vi "Clear_Lines.vi"(10 "inputArray":bool[][](array[boolean])) -> (1 "outputArray":bool[][](array[boolean]), 3 "lines":dbl)   [LabVIEW 2015]
panel:
  in  "count":dbl
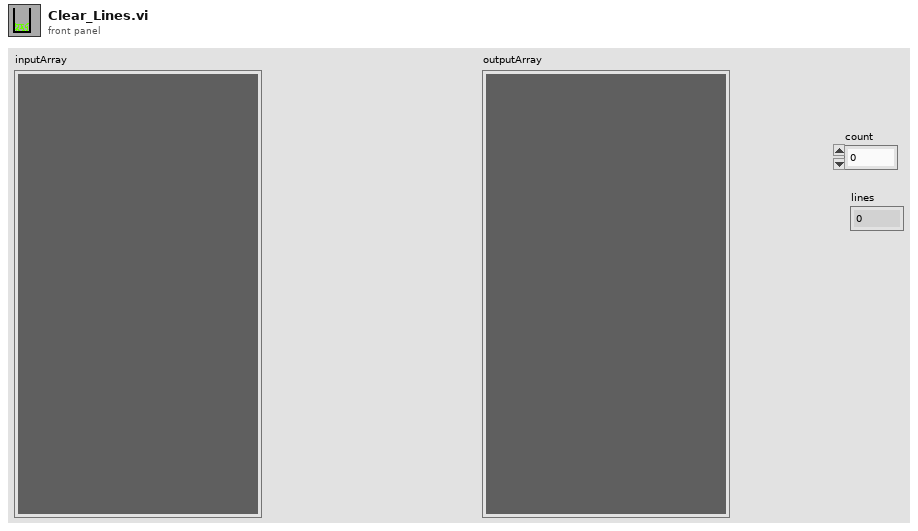
[diagram p1: front panel]
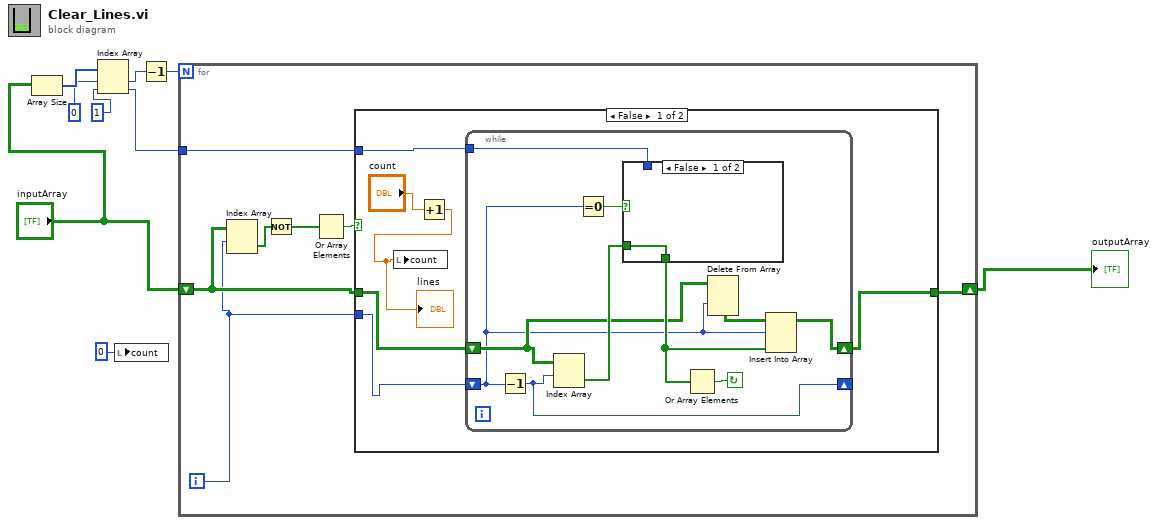
[diagram p0: block diagram]
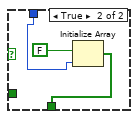
[diagram p2: hidden frame]
diagram:
  n1 = Array Size(array="inputArray") -> (size(s)=w8:i32[])
  n2 = Index Array(array=w8, index #1=0, index #2=1) -> (element #1=w6:i32, element #2=w4:i32)
  n3 = local write "count"(0) -> ()
  n4 = Decrement(x=w6) -> (x-1=w2:i32)
  n5 = for {
    N: w2 -> [_]
    shift-right: [w10] -> w3
    shift-left: "inputArray" -> [w13]
    tunnel: w4 -> [w14]
    i -> [w12]
    n6 = Index Array(array=w13, index (row)=w12) -> (element=w11:bool[])  [unwired: 1 in]
    n7 = Not(x=w11) -> (.not. x?=w16:bool[])
    n8 = Or Array Elements(Boolean array=w16) -> (logical OR=w15:bool)
    n9 = case shown="False" w15 {
      tunnel: w12 -> [w21 _]
      tunnel: w13 -> [w22 w37]
      tunnel: w14 -> [w20 _]
      tunnel: [w19 w37] -> w10
      frame False {
        n10 = Increment(x="count") -> (x+1=w17:dbl)
        "lines" <- w17
        n11 = local write "count"(w17) -> ()
        n12 = while {
          shift-right: [w31] -> _
          shift-left: w21 -> [w23]
          tunnel: w20 -> [w28]
          shift-right: [w26] -> w19
          shift-left: w22 -> [w25]
          stop <- w32 continue-if-true
          n13 = Decrement(x=w23) -> (x-1=w31:i32)
          n14 = Index Array(array=w25, index (row)=w31) -> (element=w30:bool[])  [unwired: 1 in]
          n15 = Equal To 0?(x=w23) -> (x = 0?=w29:bool)
          n16 = case shown="False" w29 {
            tunnel: w30 -> [w33 _]
            tunnel: w28 -> [_ w35]
            tunnel: [w33 w34] -> w27
            frame False {
            }
            frame True {
              n17 = Initialize Array(FALSE, w35) -> (w34:bool[])
            }
          }
          n18 = Or Array Elements(Boolean array=w27) -> (logical OR=w32:bool)
          n19 = Delete From Array(array=w25, index (row)=w23) -> (array with subset deleted=w24:bool[][])  [unwired: 2 in, 1 out]
          n20 = Insert Into Array(array=w24, index (row)=w23, new element=w27) -> (w26:bool[][])  [unwired: 1 in]
        }
      }
      frame True {
      }
    }
  }
  "outputArray" <- w3
